vi "Disconnect.vi"(8 "error in (no error)":errorcluster, 11 "CameraI2CUSB in":refnum<class "CameraSim.lvclass">) -> (0 "error out":errorcluster, 3 "CameraI2CUSB out":refnum<class "CameraSim.lvclass">)   [LabVIEW 2020, in "CameraSim.lvlib" / "CameraSim.lvclass"]
doc: "Close connection to camera"
uses:
  CameraSim.lvclass
  CameraSim.lvclass/CameraSim.ctl
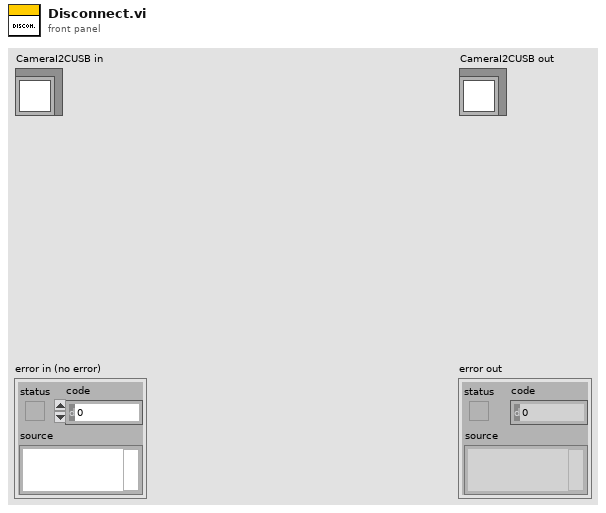
[diagram p1: front panel]
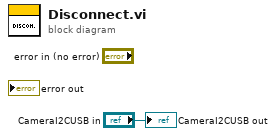
[diagram p0: block diagram]
diagram:
  "CameraI2CUSB out" <- "CameraI2CUSB in"
